vi "Send Splash Message.vi"(8 "error in (no error)":errorcluster, 10 "Message":string, 11 "Splashy":refnum<class "Splashy.lvclass">) -> (0 "error out":errorcluster, 3 "Splashy out":refnum<class "Splashy.lvclass">)   [LabVIEW 2022 SP3, in "Splashy.lvclass"]
doc: "Send a message to be display on the splash screen (adding ... at the end gives it a good touch)"
uses:
  Splashy.lvclass
  Splashy.lvclass/Splashy.ctl
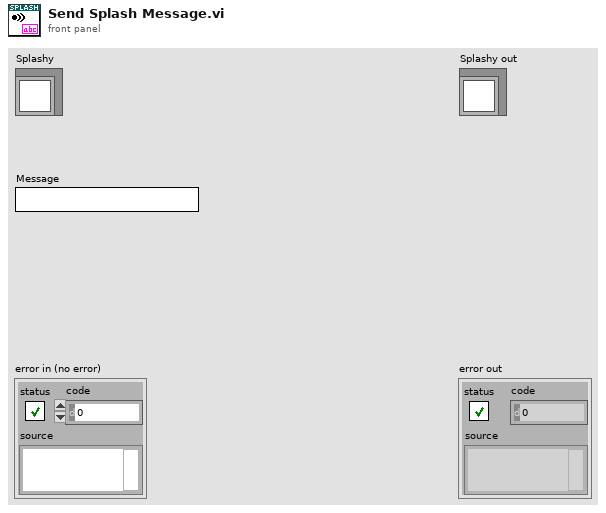
[diagram p1: front panel]
types:
  T1 = typedef "Splashy.lvclass/DisplayMessage--Cluster.ctl" = refnum<user-event>
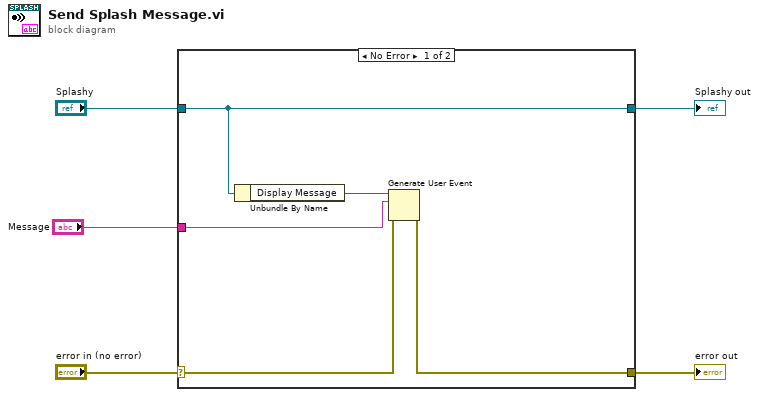
[diagram p0: block diagram]
diagram:
  n1 = case shown="No Error" "error in (no error)" {
    selector: "error in (no error)" -> [w7 w12]
    tunnel: [w6 w12] -> w4
    tunnel: [w9 w11] -> w2
    tunnel: "Splashy" -> [w9 w11]
    tunnel: "Message" -> [w8 _]
    frame No Error {
      n2 = Unbundle By Name(w9) -> ("Display Message"=w10:T1)
      n3 = Generate User Event(user event=w10, event data cluster=w8, error in=w7) -> (error out=w6:errorcluster)  [unwired: 1 in, 1 out]
    }
    frame Error {
    }
  }
  "error out" <- w4
  "Splashy out" <- w2
